vi "reshape array (AIM-1553-parameters).vi"(10 "size requested":i32=2, 11 "parameter array in":map{T1, T2[]}[](array[numeric])) -> (3 "parameter array out":map{T1, T2[]}[](array[numeric]))   [LabVIEW 2020]
uses:
  1553/_controls/1553_Parameters_key.ctl
  1553/_controls/1553_Parameters.ctl
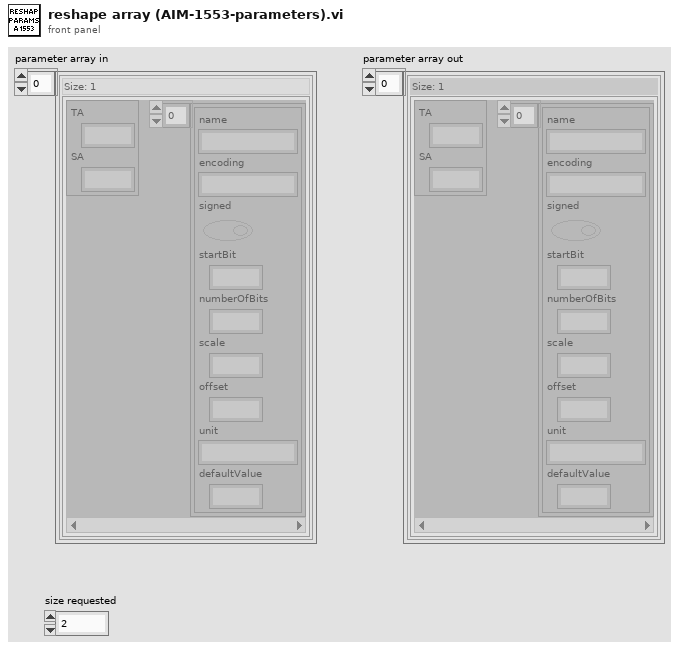
[diagram p1: front panel]
types:
  T1 = typedef "1553_Parameters_key.ctl" = cluster{"TA":i32, "SA":i32}
  T2 = typedef "1553_Parameters.ctl" = cluster{"name":string, "encoding":string, "signed":bool, "startBit":i32, "numberOfBits":i32, "scale":dbl, "offset":dbl, "unit":string, "defaultValue":dbl}
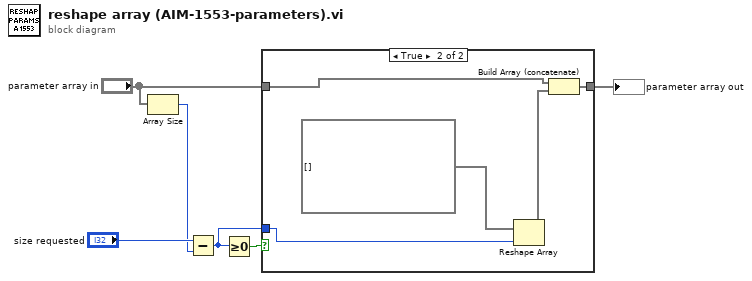
[diagram p0: block diagram]
diagram:
  n1 = Array Size(array="parameter array in") -> (size(s)=w5:i32)
  n2 = Subtract(x="size requested", y=w5) -> (x-y=w3:i32)
  n3 = Greater Or Equal To 0?(x=w3) -> (x >= 0?=w4:bool)
  n4 = case shown="True" w4 {
    tunnel: w3 -> [_ w12]
    tunnel: "parameter array in" -> [w7 w10]
    tunnel: [w7 w9] -> w1
    frame False {
    }
    frame True {
      n5 = Reshape Array(map{T1, T2[]}[] [] ("map array in 2"), w12) -> (w11:map{T1, T2[]}[])
      n6 = Build Array (concatenate)(w10, w11) -> (w9:map{T1, T2[]}[])
    }
  }
  "parameter array out" <- w1
